vi "ConnectToPannelAddressSpace.vi"(8 "error in (no error)":errorcluster, 11 "Station#":u16) -> (0 "error out":errorcluster, 3 "comms cluster":T1, 5 "local address":string, 7 "32bit local address":u32)   [LabVIEW 2025]
doc: "User gives station number. Check if \npannel is occupied. If available write\nuser id to station MB server gate register,\nif in use return error.\n\nINPUTS:\n 1. requested station id.\n\nOUTPUTS:\n 1. comms cluster of:\n a) station reg start address\n b)16-bit modulo of local user IP\n c) MB comms line \n 2. initialised error line\n 3. IP address expressed as 32-bit uint\n 4. IP address expressed as string"
uses:
  <vilib>/Modbus/master/Modbus Master.lvclass
  <vilib>/Modbus/master/Create Master Instance (TCP).vi
panel:
  # "Connect to pannel address space\n\nUser gives station number. Check if \npannel is occupied. If available write\nuser id to station MB server gate register,\nif in use return error.\n\nINPUTS:\n  1. requested station id.\n  2. initialised error line in.\nOUTPUTS:\n  1. comms cluster of:\n      a) station reg start address\n      b)16-bit modulo of local user IP\n      c) MB comms line \n   2. error line out\n   3. IP address expressed as 32-bit uint\n   4. IP address expressed as string"
  # "Station number input"
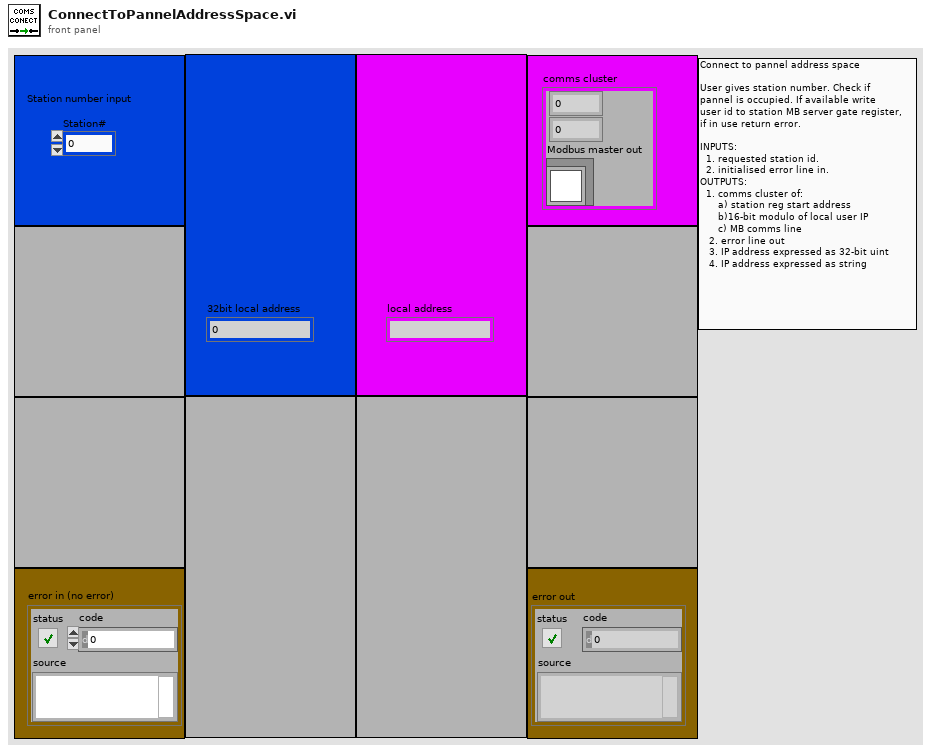
[diagram p1: front panel]
types:
  T1 = cluster{u16, u32, "Modbus master out":refnum<class "Modbus Master.lvclass">}
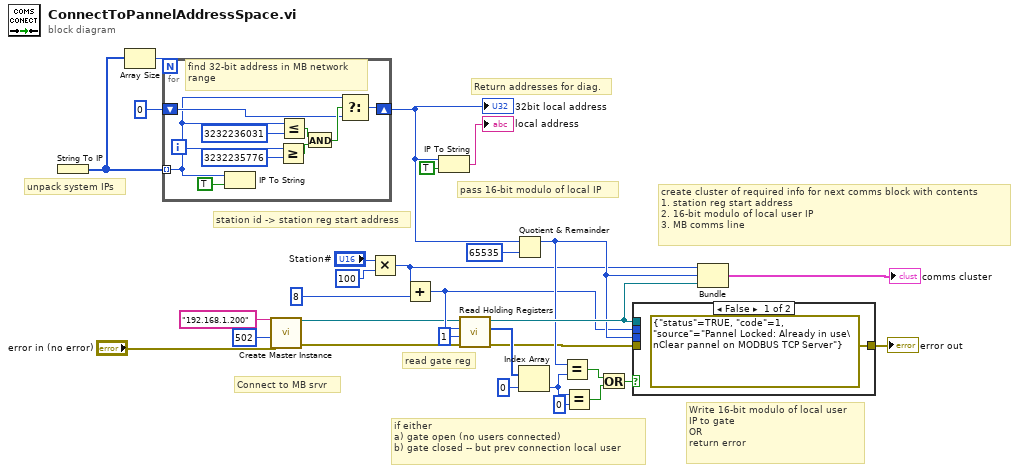
[diagram p0: block diagram]
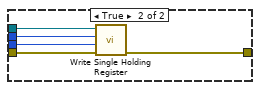
[diagram p2: hidden frame]
diagram:
  # "station id -> station reg start address"
  # "create cluster of required info for next comms block with contents\n1. station reg start address\n2. 16-bit modulo of local user IP\n3. MB comms line"
  # "pass 16-bit modulo of local IP"
  # "Write 16-bit modulo of local user\nIP to gate\nOR\nreturn error"
  # "if either\na) gate open (no users connected)\nb) gate closed -- but prev connection local user"
  # "read gate reg"
  # "Connect to MB srvr"
  # "Return addresses for diag."
  # "unpack system IPs"
  n1 = String To IP() -> (0:w5:u32[])  [unwired: 1 in]
  n2 = Array Size(array=w5) -> (size(s)=w4:i32)
  n3 = for {
    N: w4 -> [_]
    tunnel: w5 -> [w34] mode=indexing
    shift-right: [w33] -> w2
    shift-left: u32 0 ("index") -> [w35]
    # "find 32-bit address in MB network\nrange"
    n4 = IP To String(1:TRUE ("dot notation? (F)"), 2:w34) -> ()  [unwired: 1 out]
    n5 = Greater Or Equal?(x=w34, y=u32 3232235776) -> (x >= y?=w38:bool)
    n6 = Less Or Equal?(x=w34, y=u32 3232236031) -> (x <= y?=w37:bool)
    n7 = And(x=w37, y=w38) -> (x .and. y?=w36:bool)
    n8 = Select(t=w34, s=w36, f=w35) -> (s? t:f=w33:u32)
  }
  "32bit local address" <- w2
  n9 = call-poly <vilib>:"Create Master Instance.vi"("error in (no error)"="error in (no error)", "port (502)"=u16 502, "address"="192.168.1.200") -> ("error out"=w16:errorcluster, "TCP master instance"=w15:refnum<class "Modbus Master.lvclass">)  [unwired: 7 in]
  n10 = Multiply(x="Station#", y=u16 100) -> (x*y=w17:u16)
  n11 = Add(x=w17, y=u16 8) -> (x+y=w19:u16)
  n12 = IP To String(1:TRUE ("dot notation? (F)"), 2:w2) -> (0:→"local address":string)
  n13 = call-dynamic "Read Holding Registers.vi"("error in (no error)"=w16, "number of holding registers"=u16 1, "starting address"=w19, "Modbus master in"=w15) -> ("error out"=w14:errorcluster, "register values"=w21:u16[], "Modbus master out"=w27:refnum<class "Modbus Master.lvclass">)  [unwired: 5 in]
  n14 = Quotient & Remainder(x=w2, y=u32 65535) -> (x-y*floor(x/y)=w25:u32)  [unwired: 1 out]
  n15 = Index Array(array=w21, index=0) -> (element=w24:u16)
  n16 = Equal?(x=w25, y=w24) -> (x = y?=w29:bool)
  n17 = Equal?(x=w24, y=u16 0) -> (x = y?=w28:bool)
  n18 = Or(x=w29, y=w28) -> (x .or. y?=w26:bool)
  n19 = case shown="False" w26 {
    tunnel: [errorcluster {"status"=TRUE, "code"=1, "source"="Pannel Locked: Already in use\nClear pannel on MODBUS TCP Server"} ("error out") w45] -> w13
    tunnel: w27 -> [_ w44]
    tunnel: w14 -> [_ w43]
    tunnel: w19 -> [_ w42]
    tunnel: w25 -> [_ w41]
    frame False {
    }
    frame True {
      n20 = call-dynamic "Write Single Holding Register.vi"("error in (no error)"=w43, "holding register value"=w41, "address"=w42, "Modbus master in"=w44) -> ("error out"=w45:errorcluster)  [unwired: 6 in, 1 out]
    }
  }
  "error out" <- w13
  n21 = Bundle(w17, w25, "Modbus master out"=w27) -> (→"comms cluster":T1)  [unwired: 1 in]
